vi "Check For Solid.vi"(8 "error in (no error)":errorcluster, 11 "Game Engine in":refnum<class "Game Engine.lvclass">) -> (0 "error out":errorcluster, 2 "Solid Lines":i32[](array[numeric]), 3 "Game Engine out":refnum<class "Game Engine.lvclass">)   [LabVIEW 2017, in "Game Engine.lvlib" / "Game Engine.lvclass"]
uses:
  Game Engine.lvclass
  Game Engine.lvclass/Game Engine.ctl
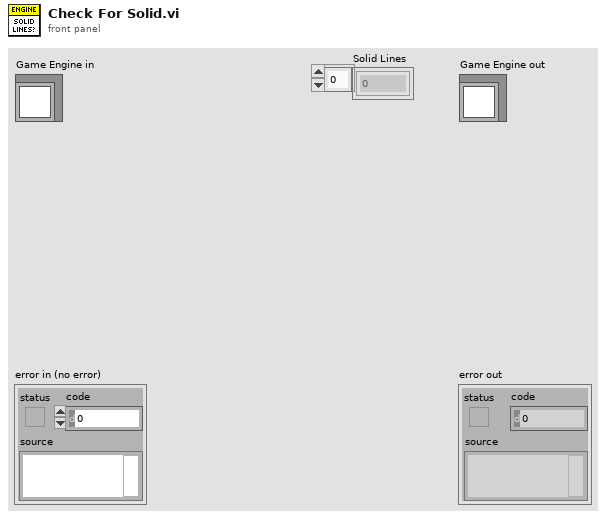
[diagram p1: front panel]
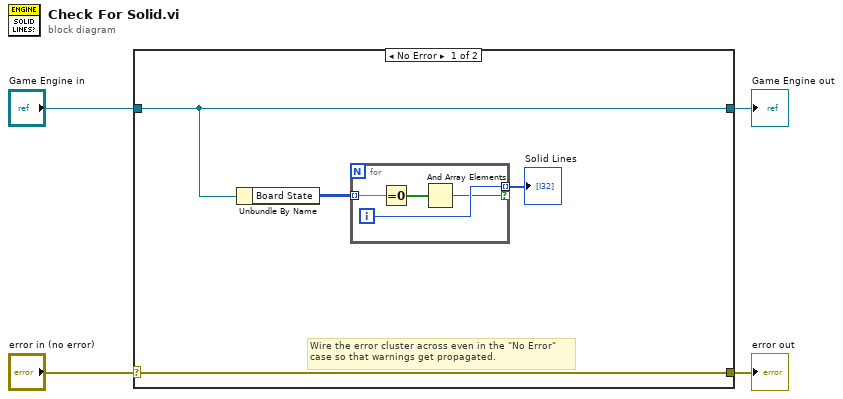
[diagram p0: block diagram]
diagram:
  n1 = case shown="No Error" "error in (no error)" {
    selector: "error in (no error)" -> [w8 w14]
    tunnel: [w8 w14] -> w3
    tunnel: [w6 w13] -> w1
    tunnel: "Game Engine in" -> [w6 w13]
    frame No Error {
      # "Wire the error cluster across even in the \"No Error\"\ncase so that warnings get propagated."
      n2 = Unbundle By Name(w6) -> ("Board State"=w7:u32[][])
      n3 = for {
        tunnel: w7 -> [w12] mode=indexing
        tunnel: [w10] -> w5 mode=indexing if=w9
        i -> [w10]
        n4 = Equal To 0?(x=w12) -> (x = 0?=w11:bool[])
        n5 = And Array Elements(Boolean array=w11) -> (logical AND=w9:bool)
      }
      "Solid Lines" <- w5
    }
    frame Error {
    }
  }
  "error out" <- w3
  "Game Engine out" <- w1
